vi "tcp_server_v2.vi"() -> ()   [LabVIEW 2019]
panel:
  out "error out":errorcluster
  out "EOS":bool=TRUE
  out "BOS":bool=TRUE
  out "server_step":i32
  out "spill_id":i32
  in  "stop_server":bool
  in  "stop_spill_inc":bool
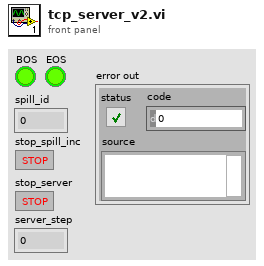
[diagram p1: front panel]
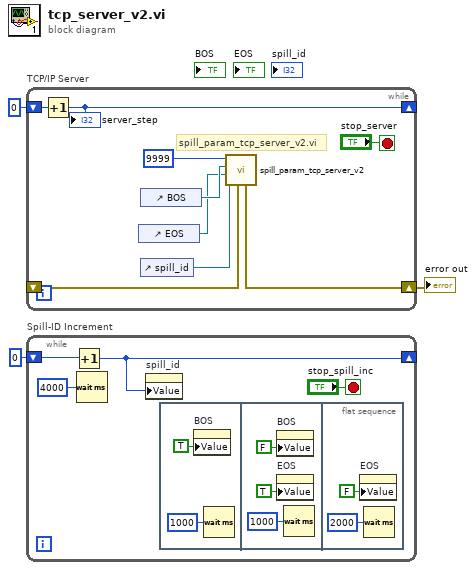
[diagram p0: block diagram]
diagram:
  n1 = while "TCP/IP Server" {
    shift-right: [w10] -> _
    shift-left: 0 -> [w11]
    shift-right: [w6] -> w1
    shift-left: _ -> [w5]
    stop <- "stop_server" stop-if-true
    # "spill_param_tcp_server_v2.vi"
    n2 = Increment(x=w11) -> (x+1=w10:i32)
    "server_step" <- w10
    n3 = control-ref of="EOS"() -> (w7:refnum<vi>)
    n4 = control-ref of="BOS"() -> (w8:refnum<vi>)
    n5 = control-ref of="spill_id"() -> (w4:refnum<vi>)
    n6 = call "spill_param_tcp_server_v2.vi"("error in"=w5, "spill_id_Refnum"=w4, "EOS_Refnum"=w7, "BOS_Refnum"=w8, "port"=u16 9999) -> ("error out"=w6:errorcluster)  [unwired: 6 in]
  }
  "error out" <- w1
  n7 = while "Spill-ID Increment" {
    shift-right: [w13] -> _
    shift-left: 0 -> [w16]
    stop <- "stop_spill_inc" stop-if-true
    n8 = Increment(x=w16) -> (x+1=w13:i32)
    n9 = Wait (ms)(milliseconds to wait=u32 4000) -> ()  [unwired: 1 out]
    n10 = property on="spill_id" class="DigNum (strict)"("Value"=w13) -> ()  [unwired: 2 in, 2 out]
    n11 = flat-sequence {
      frame #0 {
        n12 = property on="BOS" class="Bool (strict)"("Value"=TRUE) -> ()  [unwired: 2 in, 2 out]
        n13 = Wait (ms)(milliseconds to wait=u32 1000) -> ()  [unwired: 1 out]
      }
      frame #1 {
        n14 = property on="BOS" class="Bool (strict)"("Value"=FALSE) -> ()  [unwired: 2 in, 2 out]
        n15 = property on="EOS" class="Bool (strict)"("Value"=TRUE) -> ()  [unwired: 2 in, 2 out]
        n16 = Wait (ms)(milliseconds to wait=u32 1000) -> ()  [unwired: 1 out]
      }
      frame #2 {
        n17 = property on="EOS" class="Bool (strict)"("Value"=FALSE) -> ()  [unwired: 2 in, 2 out]
        n18 = Wait (ms)(milliseconds to wait=u32 2000) -> ()  [unwired: 1 out]
      }
    }
  }
